vi "FTW-Endpoint-Receive.vi"(0 "FTW Endpoint":refnum<class "FTW-Endpoint.lvclass">, 5 "Timeout":i32 format="%dmsec", 11 "error in":errorcluster) -> (4 "FTW Endpoint out":refnum<class "FTW-Endpoint.lvclass">, 6 "Message Header":string, 8 "Message Body":string, 10 "Timed out?":bool, 15 "error out":errorcluster)   [LabVIEW 2013, in "FTW-Actor.lvlib" / "FTW-Endpoint.lvclass"]
uses:
  FTW-Endpoint.lvclass
  FTW-Endpoint.lvclass/FTW-Endpoint.ctl
panel:
  # "Inputs"
  # "Outputs"
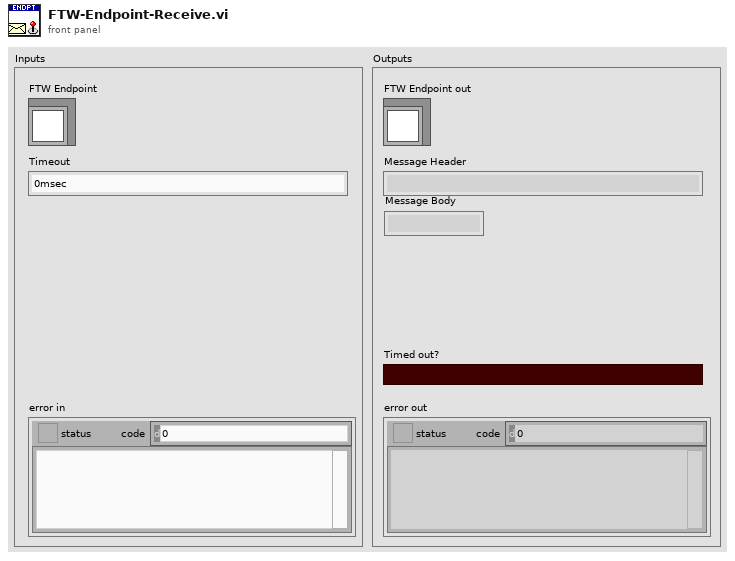
[diagram p1: front panel]
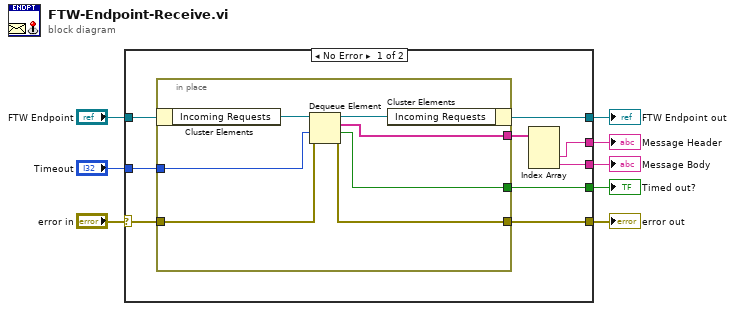
[diagram p0: block diagram]
diagram:
  n1 = case shown="No Error" "error in" {
    selector: "error in" -> [w11 w26]
    tunnel: [w10 w26] -> w8
    tunnel: [w14 w25] -> w6
    tunnel: "FTW Endpoint" -> [w15 w25]
    tunnel: [w9 _] -> w4
    tunnel: "Timeout" -> [w12 _]
    tunnel: [w17 _] -> w2
    tunnel: [w16 _] -> w1
    frame No Error {
      n2 = in-place {
        in-place-border: [w21] -> w10
        in-place-border: w11 -> [w22]
        in-place-border: w12 -> [w23]
        in-place-border: [w19] -> w13
        in-place-border: [w18] -> w9
        n3 = in-place-cluster #1(w15) -> ("Incoming Requests"=w24:refnum<queue>)
        n4 = Dequeue Element(queue=w24, timeout in ms (-1)=w23, error in (no error)=w22) -> (queue out=w20:refnum<queue>, element=w19:string[], timed out?=w18:bool, error out=w21:errorcluster)
        n5 = in-place-cluster #1("Incoming Requests"=w20) -> (w14:refnum<class "FTW-Endpoint.lvclass">)
      }
      n6 = Index Array(array=w13) -> (element #2=w17:string, element #3=w16:string)  [unwired: 3 in, 1 out]
    }
    frame Error {
    }
  }
  "error out" <- w8
  "FTW Endpoint out" <- w6
  "Timed out?" <- w4
  "Message Header" <- w2
  "Message Body" <- w1
